vi "stateClient.vi"() -> (3 "state client out":string)   [LabVIEW 2019]
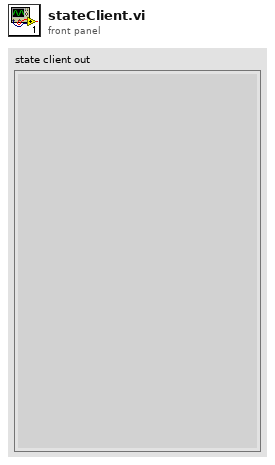
[diagram p1: front panel]
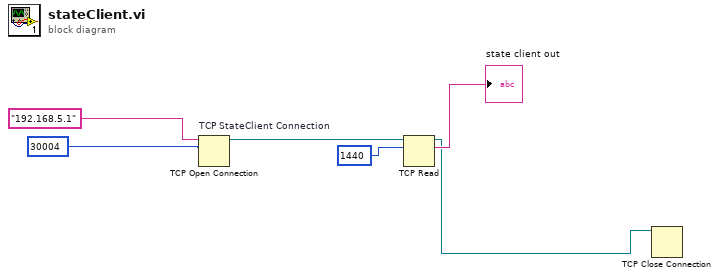
[diagram p0: block diagram]
diagram:
  n1 = TCP Open Connection "TCP StateClient Connection"(address="192.168.5.1", remote port or service name=30004) -> (connection ID=w2:refnum<k5>)  [unwired: 3 in, 1 out]
  n2 = TCP Read(connection ID=w2, bytes to read=1440) -> (connection ID out=w1:refnum<k5>, data out=→"state client out":string)  [unwired: 3 in, 1 out]
  n3 = TCP Close Connection(connection ID=w1) -> ()  [unwired: 2 in, 2 out]
